vi "get display data mini.vi"(0 "display queues":T2, 1 "prune?":bool=TRUE, 5 "time range":dbl=-1.0, 9 "t0":dbl, 11 "error in (no error)":errorcluster) -> (4 "voltage graph":cluster{dbl[], dbl[]}, 6 "coil graph":cluster{dbl[], dbl[]}, 8 "acceleration last quarter second":T1[](array[typedef]), 10 "extracted magnetism":T1[](array[typedef]), 15 "error out":errorcluster)   [LabVIEW 2017]
uses:
  typedefs/reading1.ctl
  typedefs/reading3.ctl
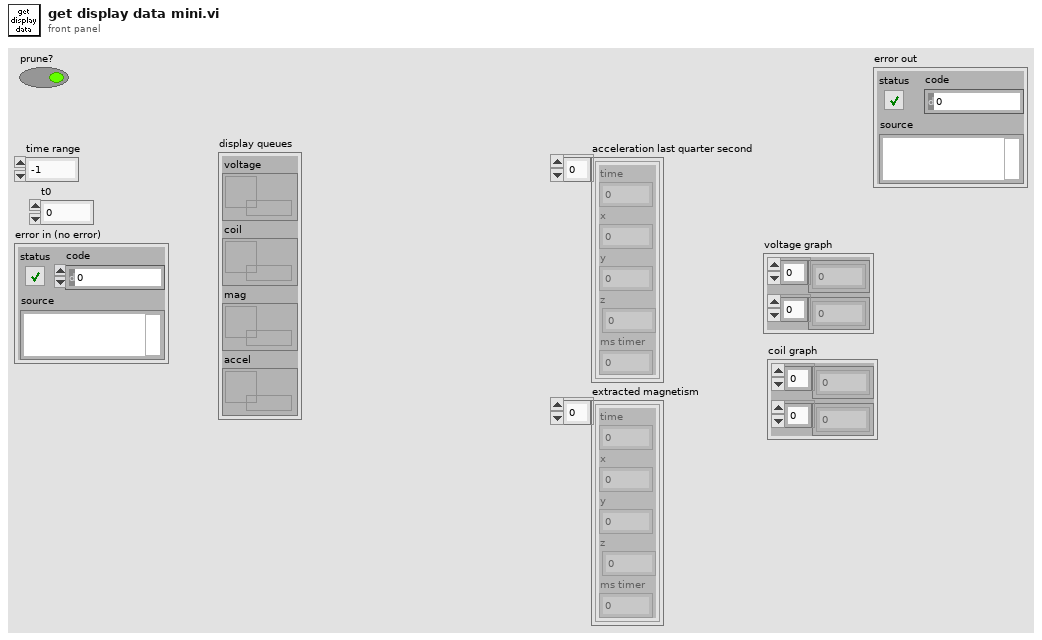
[diagram p1: front panel]
types:
  T1 = typedef "reading3.ctl" = cluster{"time":dbl, "x":dbl, "y":dbl, "z":dbl, "ms timer":u32}
  T2 = cluster{"voltage":refnum<queue>, "coil":refnum<queue>, "mag":refnum<queue>, "accel":refnum<queue>}
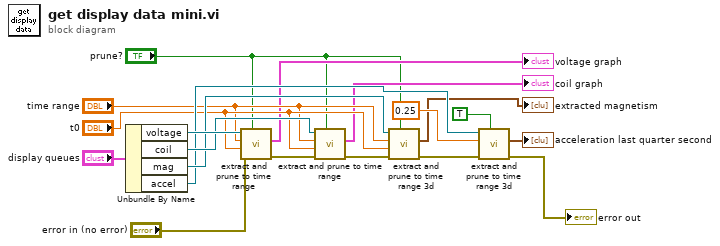
[diagram p0: block diagram]
diagram:
  n1 = Unbundle By Name("display queues") -> ("voltage"=w16:refnum<queue>, "coil"=w15:refnum<queue>, "mag"=w14:refnum<queue>, "accel"=w13:refnum<queue>)
  n2 = call "extract and prune to time range.vi"("prune?"="prune?", "error in (no error)"="error in (no error)", "t0"="t0", "time range"="time range", "time and val queue"=w16) -> ("error out"=w18:errorcluster, "graph"=→"voltage graph":cluster{dbl[], dbl[]})  [unwired: 4 in, 1 out]
  n3 = call "extract and prune to time range.vi"("prune?"="prune?", "error in (no error)"=w18, "t0"="t0", "time range"="time range", "time and val queue"=w15) -> ("error out"=w12:errorcluster, "graph"=→"coil graph":cluster{dbl[], dbl[]})  [unwired: 4 in, 1 out]
  n4 = call "extract and prune to time range 3d.vi"("prune?"="prune?", "error in (no error)"=w12, "t0"="t0", "time range"="time range", "queue in"=w14) -> ("error out"=w11:errorcluster, "extracted data"=→"extracted magnetism":T1[])  [unwired: 4 in, 1 out]
  n5 = call "extract and prune to time range 3d.vi"("prune?"=TRUE, "error in (no error)"=w11, "time range"=0.25, "queue in"=w13) -> ("error out"=→"error out":errorcluster, "extracted data"=→"acceleration last quarter second":T1[])  [unwired: 5 in, 1 out]
